vi "Process Array Elements.vi"(7 "Format String (%#0.15f)":string="%#0.15f", 8 "Error In":errorcluster, 9 "Name In":string, 10 "Array Variant":variant, 11 "Queue In":refnum<queue>) -> (0 "Error Out":errorcluster, 1 "Data Out":string, 3 "Queue Out":refnum<queue>)   [LabVIEW 2020]
doc: "This VI was created for use with the Read/Write Cluster VIs. It converts array elements of the cluster to strings to be written to file.\n\nFreeware from Moore Good Ideas, www.mooregoodideas.com. Do not remove this line."
uses:
  Koop/KObject Class/KObject.lvclass
  <vilib>/Utility/VariantDataType/VariantType.lvlib
  <vilib>/Utility/Data Type/NI_Data Type.lvlib
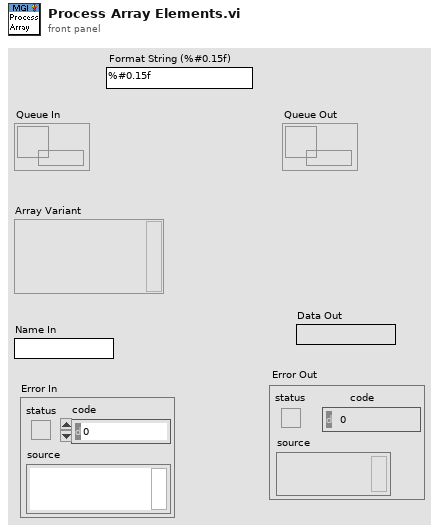
[diagram p1: front panel]
types:
  T1 = typedef "NI_Data Type.lvlib/Data Type.ctl" = enum8{"Invalid Type", "Void", "I8", "I16", "I32", "I64", "U8", "U16", "U32", "U64", "Single Float", "Double Float", "Extended Float", "Single Complex", "Double Complex", "Extended Complex", "Enum U8", "Enum U16", "Enum U32", "Enum U64", "Single Float With Unit", "Double Float With Unit", "Extended Float With Unit", "Single Complex with Unit", "Double Complex with Unit", "Extended Complex with Unit", "Boolean", "String", "Path", "Picture", "Tag", "Array", "Cluster", "Variant", "LV Variant", "Waveform", "Timestamp", "Digital Waveform", "Digital Data", "ExpressData", "Refnum", "External Data", "VI", "Poly VI", "LabVIEW Class Instance", "Fixed Point", "Set Collection", "Map Collection"}
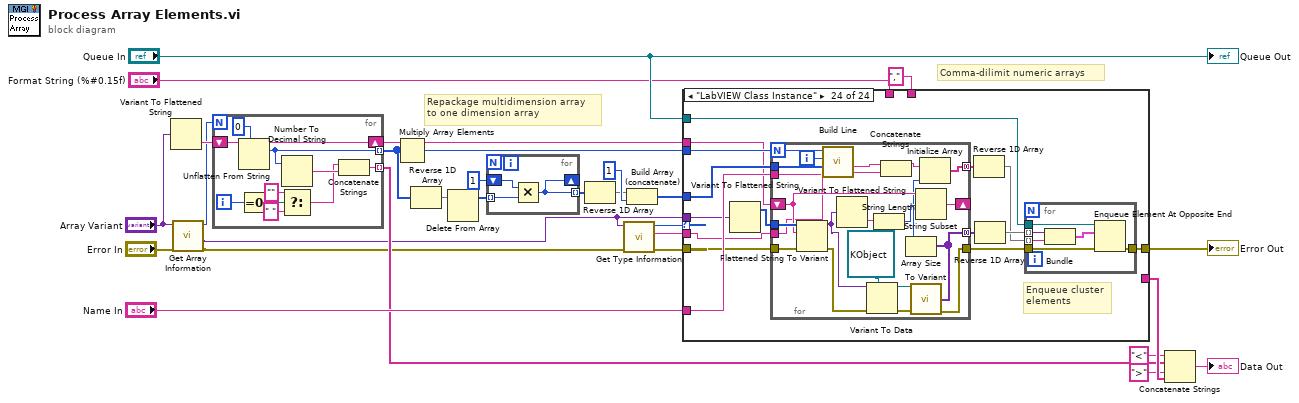
[diagram p0: block diagram]
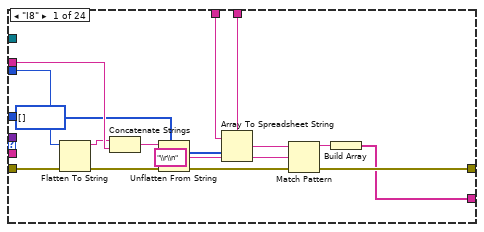
[diagram p2: hidden frame]
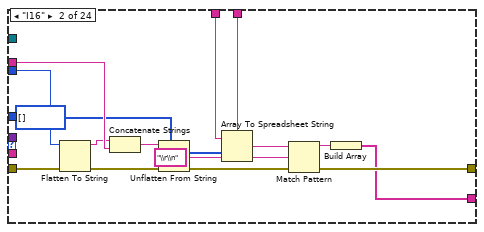
[diagram p3: hidden frame]
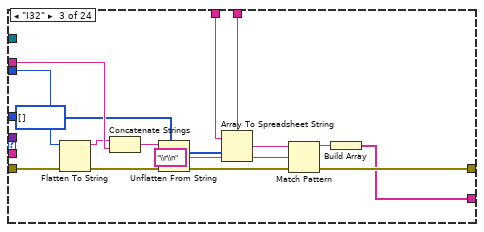
[diagram p4: hidden frame]
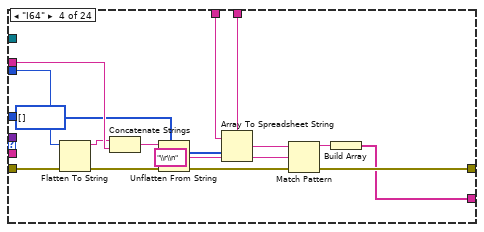
[diagram p5: hidden frame]
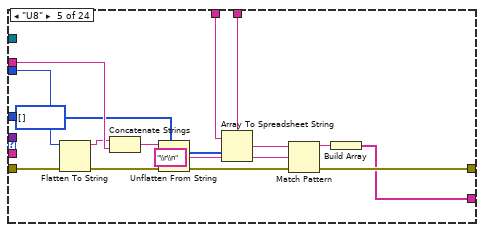
[diagram p6: hidden frame]
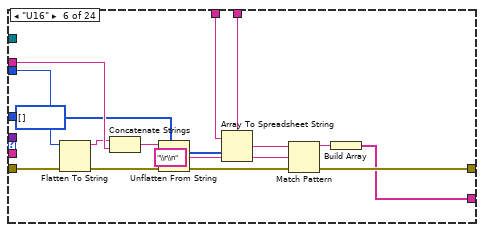
[diagram p7: hidden frame]
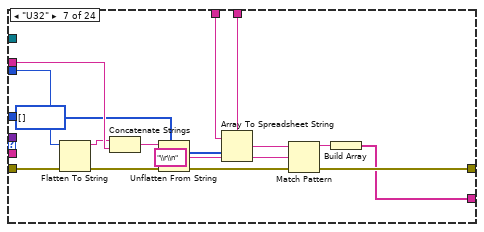
[diagram p8: hidden frame]
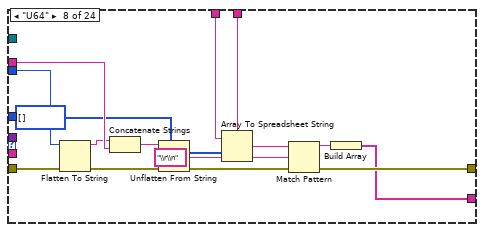
[diagram p9: hidden frame]
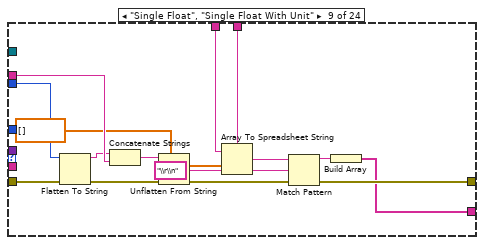
[diagram p10: hidden frame]
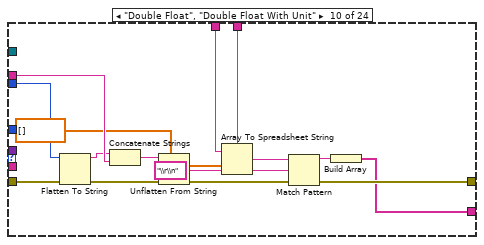
[diagram p11: hidden frame]
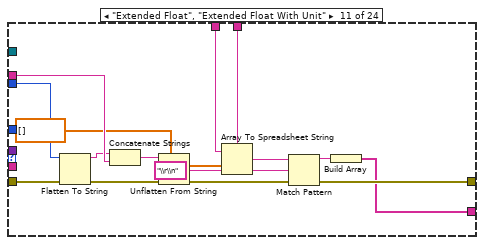
[diagram p12: hidden frame]
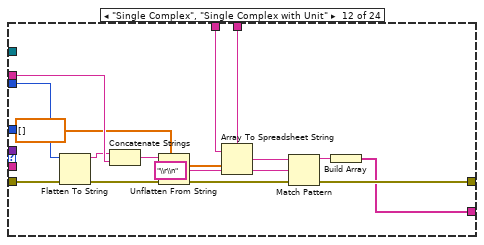
[diagram p13: hidden frame]
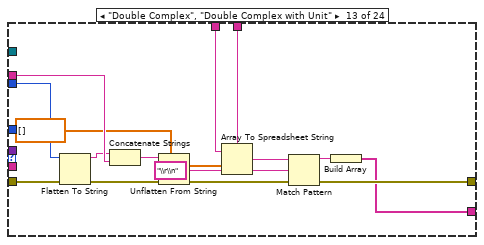
[diagram p14: hidden frame]
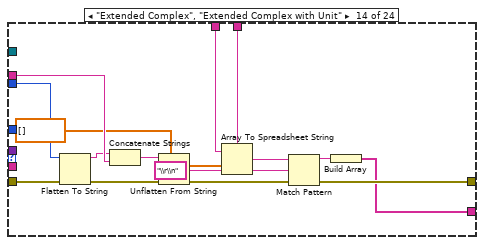
[diagram p15: hidden frame]
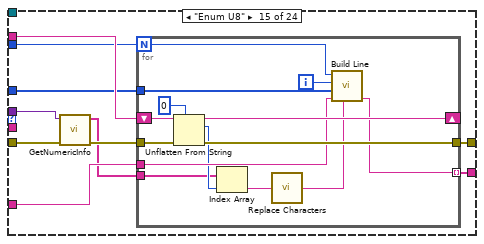
[diagram p16: hidden frame]
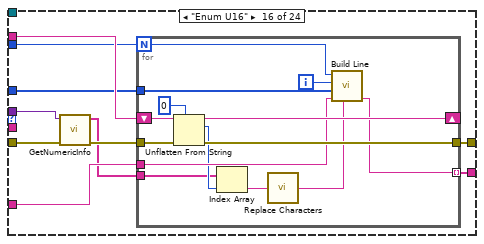
[diagram p17: hidden frame]
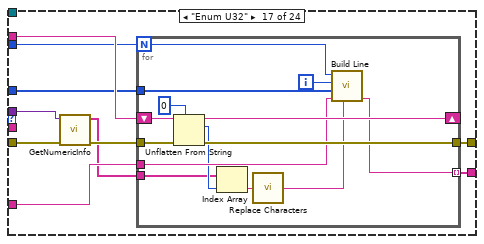
[diagram p18: hidden frame]
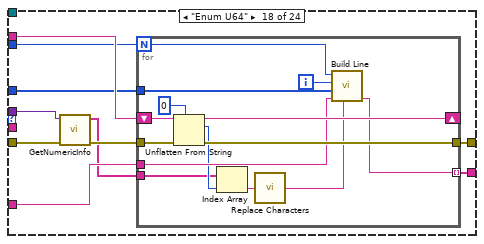
[diagram p19: hidden frame]
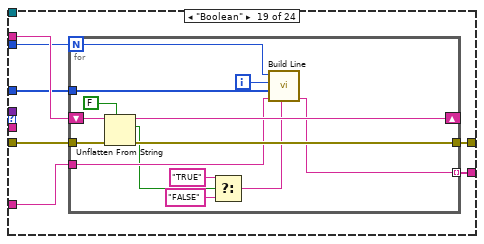
[diagram p20: hidden frame]
diagram:
  # "Comma-dilimit numeric arrays"
  # "Repackage multidimension array\nto one dimension array"
  n1 = Variant To Flattened String(Variant="Array Variant") -> (data string=w29:string)  [unwired: 1 out]
  n2 = call <vilib>:"Get Array Information.vi"("error in (no error)"="Error In", "variant"="Array Variant") -> ("error out"=w5:errorcluster, "array element data type"=w2:variant, "number of dimensions"=w4:i32)  [unwired: 6 in, 1 out]
  n3 = for {
    N: w4 -> [_]
    shift-right: [w38] -> w28
    shift-left: w29 -> [w39]
    tunnel: [w35] -> w17 mode=indexing
    tunnel: [w36] -> w13 mode=indexing
    i -> [w34]
    n4 = Unflatten From String(type=u32 0, binary string=w39) -> (rest of the binary string=w38:string, value=w35:u32)  [unwired: 3 in, 1 out]
    n5 = Equal To 0?(x=w34) -> (x = 0?=w33:bool)
    n6 = Number To Decimal String(number=w35) -> (decimal integer string=w37:string)  [unwired: 1 in]
    n7 = Select(t="", s=w33, f=" ") -> (s? t:f=w31:string)
    n8 = Concatenate Strings(w31, w37) -> (w36:string)
  }
  n9 = Multiply Array Elements(1:w17) -> (0:w27:u32)
  n10 = Reverse 1D Array(array=w17) -> (reversed array=w18:u32[])
  n11 = Delete From Array(array=w18) -> (array with subset deleted=w19:u32[])  [unwired: 2 in, 1 out]
  n12 = for {
    tunnel: w19 -> [w43] mode=indexing
    shift-right: [w41] -> _
    shift-left: i8 1 -> [w42]
    tunnel: [w41] -> w21 mode=indexing
    n13 = Multiply(x=w42, y=w43) -> (x*y=w41:u32)
  }
  n14 = Reverse 1D Array(array=w21) -> (reversed array=w22:u32[])
  n15 = call <vilib>:"Get Type Information.vi"("error in (no error)"=w5, "variant"=w2) -> ("error out"=w8:errorcluster, "name"=w1:string, "type"=w7:T1)  [unwired: 5 in, 2 out]
  n16 = Build Array (concatenate)(w22, i8 1) -> (w16:u32[])
  n17 = case shown="\"LabVIEW Class Instance\"" w7 {
    tunnel: [w58 w73 w88 w103 w118 w133 w148 w163 w178 w193 w208 w223 w238 w253 w263 w287 w311 w335 w356 w377 w396 w412 w423 w458] -> w15
    tunnel: w8 -> [w47 w62 w77 w92 w107 w122 w137 w152 w167 w182 w197 w212 w227 w242 w256 w280 w304 w328 w355 w376 w395 w412 w417 w452]
    tunnel: w28 -> [w57 w72 w87 w102 w117 w132 w147 w162 w177 w192 w207 w222 w237 w252 w262 w286 w310 w334 w354 w375 w394 w411 w419 w454]
    tunnel: w27 -> [w56 w71 w86 w101 w116 w131 w146 w161 w176 w191 w206 w221 w236 w251 w261 w285 w309 w333 w353 w374 w393 _ w430 w464]
    tunnel: "Name In" -> [_ _ _ _ _ _ _ _ _ _ _ _ _ _ w260 w284 w308 w332 w352 w373 w392 _ w429 w463]
    tunnel: [w55 w70 w85 w100 w115 w130 w145 w160 w175 w190 w205 w220 w235 w250 w258 w282 w306 w330 w350 w371 w390 w410 _ _] -> w25
    tunnel: w16 -> [_ _ _ _ _ _ _ _ _ _ _ _ _ _ w259 w283 w307 w331 w351 w372 w391 _ w428 w462]
    tunnel: "Queue In" -> [_ _ _ _ _ _ _ _ _ _ _ _ _ _ _ _ _ _ _ _ _ _ w424 w459]
    tunnel: w2 -> [_ _ _ _ _ _ _ _ _ _ _ _ _ _ w257 w281 w305 w329 _ _ _ _ w418 w453]
    tunnel: "Format String (%#0.15f)" -> [w45 w60 w75 w90 w105 w120 w135 w150 w165 w180 w195 w210 w225 w240 _ _ _ _ _ _ _ _ _ _]
    tunnel: "," ("delimiter (Tab)") -> [w44 w59 w74 w89 w104 w119 w134 w149 w164 w179 w194 w209 w224 w239 _ _ _ _ _ _ _ _ _ _]
    tunnel: w1 -> [_ _ _ _ _ _ _ _ _ _ _ _ _ _ _ _ _ _ _ _ _ _ _ w450]
    frame "I8" {
      n18 = Flatten To String(anything=w56, error in (no error)=w47) -> (data string=w52:string, error out=w46:errorcluster)  [unwired: 2 in, 1 out]
      n19 = Concatenate Strings(w52, w57) -> (w53:string)
      n20 = Unflatten From String(type=i8[] [], binary string=w53, error in (no error)=w46) -> (value=w49:i8[], error out=w58:errorcluster)  [unwired: 2 in, 1 out]
      n21 = Array To Spreadsheet String(delimiter (Tab)=w44, array=w49, 3:w45) -> (spreadsheet string=w51:string)
      n22 = Match Pattern(string=w51, regular expression="\\r\\n") -> (before substring=w48:string)  [unwired: 1 in, 3 out]
      n23 = Build Array(w48) -> (w55:string[])
    }
    frame "I16" {
      n24 = Flatten To String(anything=w71, error in (no error)=w62) -> (data string=w67:string, error out=w61:errorcluster)  [unwired: 2 in, 1 out]
      n25 = Concatenate Strings(w67, w72) -> (w68:string)
      n26 = Unflatten From String(type=i16[] [], binary string=w68, error in (no error)=w61) -> (value=w64:i16[], error out=w73:errorcluster)  [unwired: 2 in, 1 out]
      n27 = Array To Spreadsheet String(delimiter (Tab)=w59, array=w64, 3:w60) -> (spreadsheet string=w66:string)
      n28 = Match Pattern(string=w66, regular expression="\\r\\n") -> (before substring=w63:string)  [unwired: 1 in, 3 out]
      n29 = Build Array(w63) -> (w70:string[])
    }
    frame "I32" {
      n30 = Flatten To String(anything=w86, error in (no error)=w77) -> (data string=w82:string, error out=w76:errorcluster)  [unwired: 2 in, 1 out]
      n31 = Concatenate Strings(w82, w87) -> (w83:string)
      n32 = Unflatten From String(type=i32[] [], binary string=w83, error in (no error)=w76) -> (value=w79:i32[], error out=w88:errorcluster)  [unwired: 2 in, 1 out]
      n33 = Array To Spreadsheet String(delimiter (Tab)=w74, array=w79, 3:w75) -> (spreadsheet string=w81:string)
      n34 = Match Pattern(string=w81, regular expression="\\r\\n") -> (before substring=w78:string)  [unwired: 1 in, 3 out]
      n35 = Build Array(w78) -> (w85:string[])
    }
    frame "I64" {
      n36 = Flatten To String(anything=w101, error in (no error)=w92) -> (data string=w97:string, error out=w91:errorcluster)  [unwired: 2 in, 1 out]
      n37 = Concatenate Strings(w97, w102) -> (w98:string)
      n38 = Unflatten From String(type=i64[] [], binary string=w98, error in (no error)=w91) -> (value=w94:i64[], error out=w103:errorcluster)  [unwired: 2 in, 1 out]
      n39 = Array To Spreadsheet String(delimiter (Tab)=w89, array=w94, 3:w90) -> (spreadsheet string=w96:string)
      n40 = Match Pattern(string=w96, regular expression="\\r\\n") -> (before substring=w93:string)  [unwired: 1 in, 3 out]
      n41 = Build Array(w93) -> (w100:string[])
    }
    frame "U8" {
      n42 = Flatten To String(anything=w116, error in (no error)=w107) -> (data string=w112:string, error out=w106:errorcluster)  [unwired: 2 in, 1 out]
      n43 = Concatenate Strings(w112, w117) -> (w113:string)
      n44 = Unflatten From String(type=u8[] [], binary string=w113, error in (no error)=w106) -> (value=w109:u8[], error out=w118:errorcluster)  [unwired: 2 in, 1 out]
      n45 = Array To Spreadsheet String(delimiter (Tab)=w104, array=w109, 3:w105) -> (spreadsheet string=w111:string)
      n46 = Match Pattern(string=w111, regular expression="\\r\\n") -> (before substring=w108:string)  [unwired: 1 in, 3 out]
      n47 = Build Array(w108) -> (w115:string[])
    }
    frame "U16" {
      n48 = Flatten To String(anything=w131, error in (no error)=w122) -> (data string=w127:string, error out=w121:errorcluster)  [unwired: 2 in, 1 out]
      n49 = Concatenate Strings(w127, w132) -> (w128:string)
      n50 = Unflatten From String(type=u16[] [], binary string=w128, error in (no error)=w121) -> (value=w124:u16[], error out=w133:errorcluster)  [unwired: 2 in, 1 out]
      n51 = Array To Spreadsheet String(delimiter (Tab)=w119, array=w124, 3:w120) -> (spreadsheet string=w126:string)
      n52 = Match Pattern(string=w126, regular expression="\\r\\n") -> (before substring=w123:string)  [unwired: 1 in, 3 out]
      n53 = Build Array(w123) -> (w130:string[])
    }
    frame "U32" {
      n54 = Flatten To String(anything=w146, error in (no error)=w137) -> (data string=w142:string, error out=w136:errorcluster)  [unwired: 2 in, 1 out]
      n55 = Concatenate Strings(w142, w147) -> (w143:string)
      n56 = Unflatten From String(type=u32[] [], binary string=w143, error in (no error)=w136) -> (value=w139:u32[], error out=w148:errorcluster)  [unwired: 2 in, 1 out]
      n57 = Array To Spreadsheet String(delimiter (Tab)=w134, array=w139, 3:w135) -> (spreadsheet string=w141:string)
      n58 = Match Pattern(string=w141, regular expression="\\r\\n") -> (before substring=w138:string)  [unwired: 1 in, 3 out]
      n59 = Build Array(w138) -> (w145:string[])
    }
    frame "U64" {
      n60 = Flatten To String(anything=w161, error in (no error)=w152) -> (data string=w157:string, error out=w151:errorcluster)  [unwired: 2 in, 1 out]
      n61 = Concatenate Strings(w157, w162) -> (w158:string)
      n62 = Unflatten From String(type=u64[] [], binary string=w158, error in (no error)=w151) -> (value=w154:u64[], error out=w163:errorcluster)  [unwired: 2 in, 1 out]
      n63 = Array To Spreadsheet String(delimiter (Tab)=w149, array=w154, 3:w150) -> (spreadsheet string=w156:string)
      n64 = Match Pattern(string=w156, regular expression="\\r\\n") -> (before substring=w153:string)  [unwired: 1 in, 3 out]
      n65 = Build Array(w153) -> (w160:string[])
    }
    frame "Single Float", "Single Float With Unit" {
      n66 = Flatten To String(anything=w176, error in (no error)=w167) -> (data string=w172:string, error out=w166:errorcluster)  [unwired: 2 in, 1 out]
      n67 = Concatenate Strings(w172, w177) -> (w173:string)
      n68 = Unflatten From String(type=sgl[] [], binary string=w173, error in (no error)=w166) -> (value=w169:sgl[], error out=w178:errorcluster)  [unwired: 2 in, 1 out]
      n69 = Array To Spreadsheet String(delimiter (Tab)=w164, array=w169, 3:w165) -> (spreadsheet string=w171:string)
      n70 = Match Pattern(string=w171, regular expression="\\r\\n") -> (before substring=w168:string)  [unwired: 1 in, 3 out]
      n71 = Build Array(w168) -> (w175:string[])
    }
    frame "Double Float", "Double Float With Unit" {
      n72 = Flatten To String(anything=w191, error in (no error)=w182) -> (data string=w187:string, error out=w181:errorcluster)  [unwired: 2 in, 1 out]
      n73 = Concatenate Strings(w187, w192) -> (w188:string)
      n74 = Unflatten From String(type=dbl[] [], binary string=w188, error in (no error)=w181) -> (value=w184:dbl[], error out=w193:errorcluster)  [unwired: 2 in, 1 out]
      n75 = Array To Spreadsheet String(delimiter (Tab)=w179, array=w184, 3:w180) -> (spreadsheet string=w186:string)
      n76 = Match Pattern(string=w186, regular expression="\\r\\n") -> (before substring=w183:string)  [unwired: 1 in, 3 out]
      n77 = Build Array(w183) -> (w190:string[])
    }
    frame "Extended Float", "Extended Float With Unit" {
      n78 = Flatten To String(anything=w206, error in (no error)=w197) -> (data string=w202:string, error out=w196:errorcluster)  [unwired: 2 in, 1 out]
      n79 = Concatenate Strings(w202, w207) -> (w203:string)
      n80 = Unflatten From String(type=ext[] [], binary string=w203, error in (no error)=w196) -> (value=w199:ext[], error out=w208:errorcluster)  [unwired: 2 in, 1 out]
      n81 = Array To Spreadsheet String(delimiter (Tab)=w194, array=w199, 3:w195) -> (spreadsheet string=w201:string)
      n82 = Match Pattern(string=w201, regular expression="\\r\\n") -> (before substring=w198:string)  [unwired: 1 in, 3 out]
      n83 = Build Array(w198) -> (w205:string[])
    }
    frame "Single Complex", "Single Complex with Unit" {
      n84 = Flatten To String(anything=w221, error in (no error)=w212) -> (data string=w217:string, error out=w211:errorcluster)  [unwired: 2 in, 1 out]
      n85 = Concatenate Strings(w217, w222) -> (w218:string)
      n86 = Unflatten From String(type=csg[] [], binary string=w218, error in (no error)=w211) -> (value=w214:csg[], error out=w223:errorcluster)  [unwired: 2 in, 1 out]
      n87 = Array To Spreadsheet String(delimiter (Tab)=w209, array=w214, 3:w210) -> (spreadsheet string=w216:string)
      n88 = Match Pattern(string=w216, regular expression="\\r\\n") -> (before substring=w213:string)  [unwired: 1 in, 3 out]
      n89 = Build Array(w213) -> (w220:string[])
    }
    frame "Double Complex", "Double Complex with Unit" {
      n90 = Flatten To String(anything=w236, error in (no error)=w227) -> (data string=w232:string, error out=w226:errorcluster)  [unwired: 2 in, 1 out]
      n91 = Concatenate Strings(w232, w237) -> (w233:string)
      n92 = Unflatten From String(type=cdb[] [], binary string=w233, error in (no error)=w226) -> (value=w229:cdb[], error out=w238:errorcluster)  [unwired: 2 in, 1 out]
      n93 = Array To Spreadsheet String(delimiter (Tab)=w224, array=w229, 3:w225) -> (spreadsheet string=w231:string)
      n94 = Match Pattern(string=w231, regular expression="\\r\\n") -> (before substring=w228:string)  [unwired: 1 in, 3 out]
      n95 = Build Array(w228) -> (w235:string[])
    }
    frame "Extended Complex", "Extended Complex with Unit" {
      n96 = Flatten To String(anything=w251, error in (no error)=w242) -> (data string=w247:string, error out=w241:errorcluster)  [unwired: 2 in, 1 out]
      n97 = Concatenate Strings(w247, w252) -> (w248:string)
      n98 = Unflatten From String(type=cxt[] [], binary string=w248, error in (no error)=w241) -> (value=w244:cxt[], error out=w253:errorcluster)  [unwired: 2 in, 1 out]
      n99 = Array To Spreadsheet String(delimiter (Tab)=w239, array=w244, 3:w240) -> (spreadsheet string=w246:string)
      n100 = Match Pattern(string=w246, regular expression="\\r\\n") -> (before substring=w243:string)  [unwired: 1 in, 3 out]
      n101 = Build Array(w243) -> (w250:string[])
    }
    frame "Enum U8" {
      n102 = call <vilib>:"GetNumericInfo.vi"("error in (no error)"=w256, "Variant"=w257) -> ("error out"=w255:errorcluster, "EnumNames"=w254:string[])  [unwired: 6 in, 2 out]
      n103 = for {
        N: w261 -> [w273]
        tunnel: [w274] -> w263
        tunnel: w255 -> [w275]
        shift-right: [w276] -> _
        shift-left: w262 -> [w277]
        tunnel: w260 -> [w269]
        tunnel: [w270] -> w258 mode=indexing
        tunnel: w259 -> [w271]
        tunnel: w254 -> [w266]
        i -> [w272]
        n104 = Unflatten From String(type=u8 0, binary string=w277, error in (no error)=w275) -> (rest of the binary string=w276:string, value=w267:u8, error out=w274:errorcluster)  [unwired: 2 in]
        n105 = Index Array(array=w266, index=w267) -> (element=w265:string)
        n106 = call "Replace Characters.vi"("String In"=w265) -> ("String Out"=w264:string)  [unwired: 1 in]
        n107 = call "Build Line.vi"("Value String (\"\")"=w264, "Name In"=w269, "Array"=w271, "Iteration"=w272, "Iterations"=w273) -> ("Line"=w270:string)  [unwired: 5 in, 1 out]
      }
    }
    frame "Enum U16" {
      n108 = call <vilib>:"GetNumericInfo.vi"("error in (no error)"=w280, "Variant"=w281) -> ("error out"=w279:errorcluster, "EnumNames"=w278:string[])  [unwired: 6 in, 2 out]
      n109 = for {
        N: w285 -> [w297]
        tunnel: [w298] -> w287
        tunnel: w279 -> [w299]
        shift-right: [w300] -> _
        shift-left: w286 -> [w301]
        tunnel: w284 -> [w293]
        tunnel: [w294] -> w282 mode=indexing
        tunnel: w283 -> [w295]
        tunnel: w278 -> [w290]
        i -> [w296]
        n110 = Unflatten From String(type=u16 0, binary string=w301, error in (no error)=w299) -> (rest of the binary string=w300:string, value=w291:u16, error out=w298:errorcluster)  [unwired: 2 in]
        n111 = Index Array(array=w290, index=w291) -> (element=w289:string)
        n112 = call "Replace Characters.vi"("String In"=w289) -> ("String Out"=w288:string)  [unwired: 1 in]
        n113 = call "Build Line.vi"("Value String (\"\")"=w288, "Name In"=w293, "Array"=w295, "Iteration"=w296, "Iterations"=w297) -> ("Line"=w294:string)  [unwired: 5 in, 1 out]
      }
    }
    frame "Enum U32" {
      n114 = call <vilib>:"GetNumericInfo.vi"("error in (no error)"=w304, "Variant"=w305) -> ("error out"=w303:errorcluster, "EnumNames"=w302:string[])  [unwired: 6 in, 2 out]
      n115 = for {
        N: w309 -> [w321]
        tunnel: [w322] -> w311
        tunnel: w303 -> [w323]
        shift-right: [w324] -> _
        shift-left: w310 -> [w325]
        tunnel: w308 -> [w317]
        tunnel: [w318] -> w306 mode=indexing
        tunnel: w307 -> [w319]
        tunnel: w302 -> [w314]
        i -> [w320]
        n116 = Unflatten From String(type=u32 0, binary string=w325, error in (no error)=w323) -> (rest of the binary string=w324:string, value=w315:u32, error out=w322:errorcluster)  [unwired: 2 in]
        n117 = Index Array(array=w314, index=w315) -> (element=w313:string)
        n118 = call "Replace Characters.vi"("String In"=w313) -> ("String Out"=w312:string)  [unwired: 1 in]
        n119 = call "Build Line.vi"("Value String (\"\")"=w312, "Name In"=w317, "Array"=w319, "Iteration"=w320, "Iterations"=w321) -> ("Line"=w318:string)  [unwired: 5 in, 1 out]
      }
    }
    frame "Enum U64" {
      n120 = call <vilib>:"GetNumericInfo.vi"("error in (no error)"=w328, "Variant"=w329) -> ("error out"=w327:errorcluster, "EnumNames"=w326:string[])  [unwired: 6 in, 2 out]
      n121 = for {
        N: w333 -> [w345]
        tunnel: [w346] -> w335
        tunnel: w327 -> [w347]
        shift-right: [w348] -> _
        shift-left: w334 -> [w349]
        tunnel: w332 -> [w341]
        tunnel: [w342] -> w330 mode=indexing
        tunnel: w331 -> [w343]
        tunnel: w326 -> [w338]
        i -> [w344]
        n122 = Unflatten From String(type=u64 0, binary string=w349, error in (no error)=w347) -> (rest of the binary string=w348:string, value=w339:u64, error out=w346:errorcluster)  [unwired: 2 in]
        n123 = Index Array(array=w338, index=w339) -> (element=w337:string)
        n124 = call "Replace Characters.vi"("String In"=w337) -> ("String Out"=w336:string)  [unwired: 1 in]
        n125 = call "Build Line.vi"("Value String (\"\")"=w336, "Name In"=w341, "Array"=w343, "Iteration"=w344, "Iterations"=w345) -> ("Line"=w342:string)  [unwired: 5 in, 1 out]
      }
    }
    frame "Boolean" {
      n126 = for {
        N: w353 -> [w366]
        tunnel: [w367] -> w356
        tunnel: w355 -> [w368]
        shift-right: [w369] -> _
        shift-left: w354 -> [w370]
        tunnel: w352 -> [w362]
        tunnel: [w363] -> w350 mode=indexing
        tunnel: w351 -> [w364]
        i -> [w365]
        n127 = Unflatten From String(type=FALSE, binary string=w370, error in (no error)=w368) -> (rest of the binary string=w369:string, value=w358:bool, error out=w367:errorcluster)  [unwired: 2 in]
        n128 = Select(t="TRUE", s=w358, f="FALSE") -> (s? t:f=w357:string)
        n129 = call "Build Line.vi"("Value String (\"\")"=w357, "Name In"=w362, "Array"=w364, "Iteration"=w365, "Iterations"=w366) -> ("Line"=w363:string)  [unwired: 5 in, 1 out]
      }
    }
    frame "String" {
      n130 = for {
        N: w374 -> [w385]
        tunnel: [w386] -> w377
        tunnel: w376 -> [w387]
        shift-right: [w388] -> _
        shift-left: w375 -> [w389]
        tunnel: w373 -> [w381]
        tunnel: [w382] -> w371 mode=indexing
        tunnel: w372 -> [w383]
        i -> [w384]
        n131 = Unflatten From String(type="", binary string=w389, error in (no error)=w387) -> (rest of the binary string=w388:string, value=w379:string, error out=w386:errorcluster)  [unwired: 2 in]
        n132 = call "Replace Characters.vi"("String In"=w379) -> ("String Out"=w378:string)  [unwired: 1 in]
        n133 = call "Build Line.vi"("Value String (\"\")"=w378, "Name In"=w381, "Array"=w383, "Iteration"=w384, "Iterations"=w385) -> ("Line"=w382:string)  [unwired: 5 in, 1 out]
      }
    }
    frame "Path" {
      n134 = for {
        N: w393 -> [w405]
        tunnel: [w406] -> w396
        tunnel: w395 -> [w407]
        shift-right: [w408] -> _
        shift-left: w394 -> [w409]
        tunnel: w392 -> [w401]
        tunnel: [w402] -> w390 mode=indexing
        tunnel: w391 -> [w403]
        i -> [w404]
        n135 = Unflatten From String(type=path "", binary string=w409, error in (no error)=w407) -> (rest of the binary string=w408:string, value=w399:path, error out=w406:errorcluster)  [unwired: 2 in]
        n136 = Path To String(path=w399) -> (string=w398:string)
        n137 = call "Replace Characters.vi"("String In"=w398) -> ("String Out"=w397:string)  [unwired: 1 in]
        n138 = call "Build Line.vi"("Value String (\"\")"=w397, "Name In"=w401, "Array"=w403, "Iteration"=w404, "Iterations"=w405) -> ("Line"=w402:string)  [unwired: 5 in, 1 out]
      }
    }
    frame Default {
      n139 = String To Byte Array(string=w411) -> (unsigned byte array=w416:u8[])
      n140 = Number To Hexadecimal String(1:i16 2 ("width (-)"), 2:w416) -> (0:w415:string[])
      n141 = Build Array (concatenate)("0x", w415) -> (w410:string[])
    }
    frame "Cluster" {
      # "Enqueue cluster\nelements"
      n142 = Variant To Flattened String(Variant=w418) -> (1:w421:i16[])  [unwired: 1 out]
      n143 = for {
        N: w430 -> [w449]
        tunnel: [w443] -> w425
        tunnel: w417 -> [w445]
        tunnel: w429 -> [w441]
        tunnel: w428 -> [w447]
        tunnel: [w437] -> w426 mode=indexing
        tunnel: [w446] -> w422 mode=indexing
        tunnel: w421 -> [w444]
        shift-right: [w438] -> _
        shift-left: w419 -> [w439]
        i -> [w448]
        n144 = Flattened String To Variant(4:w445, 6:w439, 7:w444) -> (0:w443:errorcluster, 3:w437:variant)
        n145 = Variant To Flattened String(Variant=w437) -> (data string=w442:string)  [unwired: 1 out]
        n146 = String Length(string=w442) -> (length=w440:i32)
        n147 = String Subset(string=w439, offset (0)=w440) -> (substring=w438:string)  [unwired: 1 in]
        n148 = call "Build Line.vi"("Name In"=w441, "Array"=w447, "Iteration"=w448, "Iterations"=w449) -> ("Name Out"=w446:string)  [unwired: 6 in, 1 out]
      }
      n149 = Reverse 1D Array(array=w422) -> (reversed array=w420:string[])
      n150 = Reverse 1D Array(array=w426) -> (reversed array=w427:variant[])
      n151 = for {
        tunnel: [w436] -> w423
        tunnel: w427 -> [w435] mode=indexing
        tunnel: w425 -> [w434]
        tunnel: w424 -> [w432]
        tunnel: w420 -> [w431] mode=indexing
        n152 = Bundle("Variant"=w435, "Name Out"=w431) -> (w433:cluster{"Variant":variant, "Name Out":string})  [unwired: 1 in]
        n153 = Enqueue Element At Opposite End(queue=w432, element=w433, error in (no error)=w434) -> (error out=w436:errorcluster)  [unwired: 1 in, 2 out]
      }
    }
    frame "LabVIEW Class Instance" {
      # "Enqueue cluster\nelements"
      n154 = Variant To Flattened String(Variant=w453) -> (1:w456:i16[])  [unwired: 1 out]
      n155 = for {
        N: w464 -> [w492]
        tunnel: [w479] -> w460
        tunnel: w452 -> [w489]
        tunnel: w463 -> [w473]
        tunnel: w462 -> [w490]
        tunnel: [w475] -> w451 mode=concatenating
        tunnel: [w477] -> w457 mode=concatenating
        tunnel: w456 -> [w488]
        shift-right: [w484] -> _
        shift-left: w454 -> [w485]
        tunnel: w450 -> [w474]
        i -> [w491]
        n156 = Flattened String To Variant(4:w489, 6:w485, 7:w488) -> (0:w480:errorcluster, 3:w478:variant)
        n157 = call "Build Line.vi"("Name In"=w473, "Array"=w490, "Iteration"=w491, "Iterations"=w492) -> ("Name Out"=w472:string)  [unwired: 6 in, 1 out]
        n158 = Variant To Flattened String(Variant=w478) -> (data string=w487:string)  [unwired: 1 out]
        n159 = Variant To Data(error in=w480, type=refnum<class "KObject.lvclass"> refnum ("KObject"), Variant=w478) -> (data=w482:refnum<class "KObject.lvclass">, error out=w481:errorcluster)
        n160 = String Length(string=w487) -> (length=w486:i32)
        n161 = Concatenate Strings(w472, w474) -> (w471:string)
        n162 = call-dynamic "To Variant.vi"("KObject in"=w482, "error in (no error)"=w481) -> ("Array"=w475:variant[], "error out"=w479:errorcluster)  [unwired: 11 in, 1 out]
        n163 = Array Size(array=w475) -> (size(s)=w476:i32)
        n164 = String Subset(string=w485, offset (0)=w486) -> (substring=w484:string)  [unwired: 1 in]
        n165 = Initialize Array(w471, w476) -> (w477:string[])
      }
      n166 = Reverse 1D Array(array=w457) -> (reversed array=w455:string[])
      n167 = Reverse 1D Array(array=w451) -> (reversed array=w461:variant[])
      n168 = for {
        tunnel: [w470] -> w458
        tunnel: w461 -> [w469] mode=indexing
        tunnel: w460 -> [w468]
        tunnel: w459 -> [w466]
        tunnel: w455 -> [w465] mode=indexing
        n169 = Bundle("Variant"=w469, w465) -> (w467:cluster{"Variant":variant, string})  [unwired: 1 in]
        n170 = Enqueue Element At Opposite End(queue=w466, element=w467, error in (no error)=w468) -> (error out=w470:errorcluster)  [unwired: 1 in, 2 out]
      }
    }
  }
  "Error Out" <- w15
  n171 = Concatenate Strings("<", w13, ">", w25) -> (→"Data Out":string)
  "Queue Out" <- "Queue In"
